vi "STAT.vi"(8 "error in (no error)":errorcluster, 11 "FTP in":refnum<class "FTP.lvclass">) -> (0 "error out":errorcluster, 2 "status":string, 3 "FTP out":refnum<class "FTP.lvclass">)   [LabVIEW 2017, in "FTP.lvlib" / "FTP.lvclass"]
uses:
  FTP.lvclass
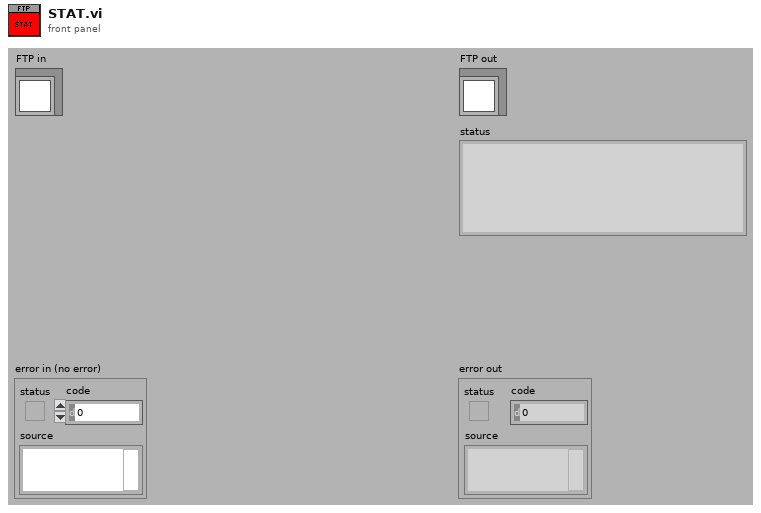
[diagram p1: front panel]
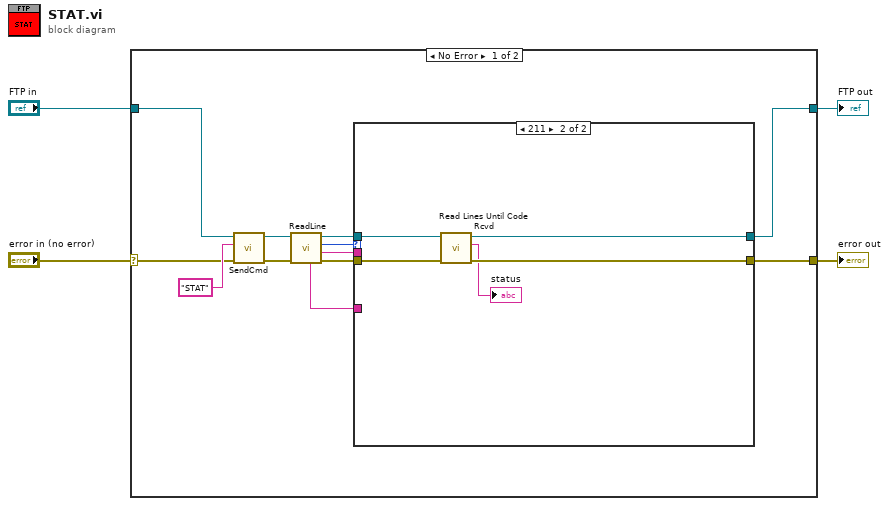
[diagram p0: block diagram]
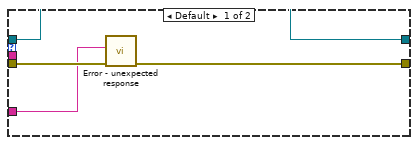
[diagram p2: hidden frame]
diagram:
  n1 = case shown="No Error" "error in (no error)" {
    selector: "error in (no error)" -> [w14 w27]
    tunnel: [w12 w27] -> w3
    tunnel: [w13 w26] -> w1
    tunnel: "FTP in" -> [w15 w26]
    frame No Error {
      n2 = call "SendCmd.vi"("error in (no error)"=w14, "cmd"="STAT", "FTP in"=w15) -> ("error out"=w11:errorcluster, "FTP out"=w10:refnum<class "FTP.lvclass">)  [unwired: 7 in]
      n3 = call "ReadLine.vi"("error in (no error)"=w11, "FTP in"=w10) -> ("error out"=w8:errorcluster, "Line"=w6:string, "code"=w7:i32, "FTP out"=w9:refnum<class "FTP.lvclass">, "Full Line"=w5:string)  [unwired: 5 in]
      n4 = case shown="211" w7 {
        tunnel: [w20 w23] -> w13
        tunnel: [w18 w22] -> w12
        tunnel: w9 -> [w20 w25]
        tunnel: w8 -> [w19 w24]
        tunnel: w6 -> [_ _]
        tunnel: w5 -> [w17 _]
        frame Default {
          n5 = call "Error - unexpected response.vi"("error in (no error)"=w19, "Full Response"=w17) -> ("error out"=w18:errorcluster)  [unwired: 9 in]
        }
        frame 211 {
          n6 = call "Read Lines Until Code Rcvd.vi"("error in (no error)"=w24, "FTP in"=w25) -> ("error out"=w22:errorcluster, "String"=→"status":string, "FTP out"=w23:refnum<class "FTP.lvclass">)  [unwired: 7 in]
        }
      }
    }
    frame Error {
    }
  }
  "error out" <- w3
  "FTP out" <- w1
